vi "DAQ setting.vi"(8 "error in (no error)":errorcluster, 11 "vi reference":refnum<vi>) -> (0 "error Out":errorcluster, 3 "Out reference":refnum<vi>)   [LabVIEW 2015]
uses:
  Control Button/Exit.ctl
  Control Button/Save.ctl
  <vilib>/addons/database/Connection.llb/DB Tools Open Connec (String).vi
  <vilib>/addons/database/_DB Variant To Data/Database Variant To Data.xnode
  <vilib>/addons/database/NI_Database_API.lvlib
panel:
  out "error out":errorcluster
  in  "read":bool
  out "subarray":string[](array[string])
  in  "Save":T1
  in  "Exit":T2
  in  "Tab Control":T3(tab)
  in  "DAQmx OutPut Setting":T4
  in  "DAQmx InPut Setting":T5
  in  "DAQmx Analog Input Setting":T6
  in  "DAQmx  Counter In":tag
  in  "DAQmx  Counter In":tag
  in  "DAQmx Counter Out":tag
  # "Digital Output  Configuration"
  # "Digital Input Configuration"
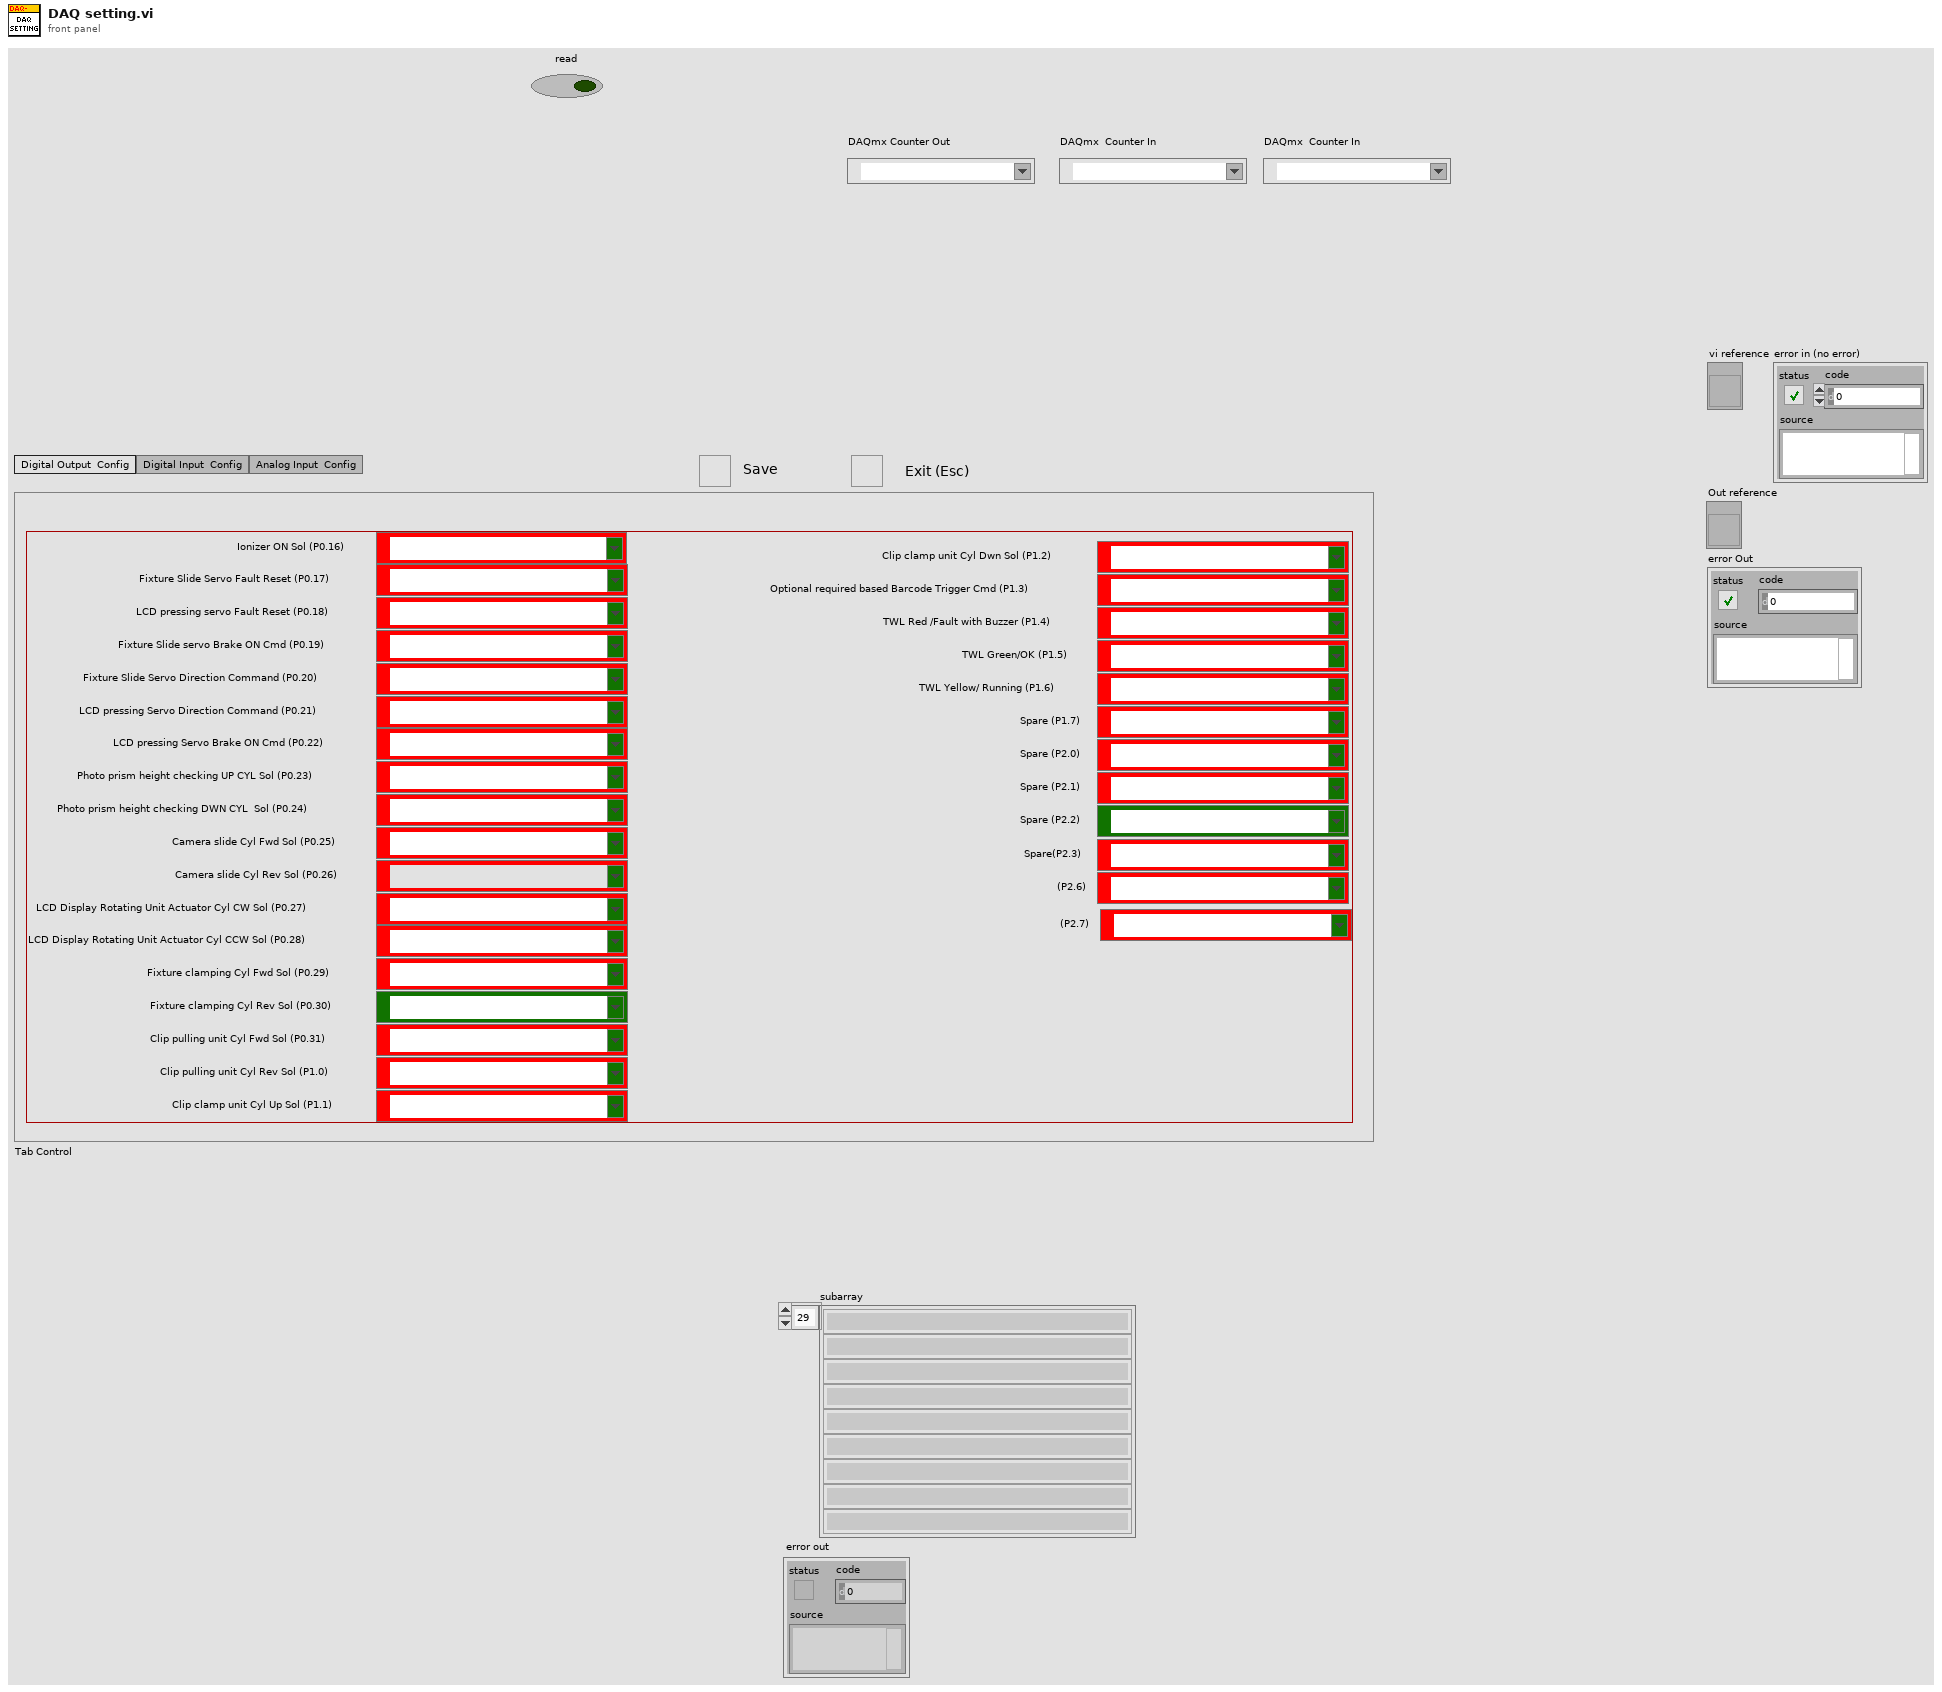
[diagram p1: front panel]
types:
  T1 = typedef "Save.ctl" = bool
  T2 = typedef "Exit.ctl" = bool
  T3 = enum32{"Digital Output  Config", "Digital Input  Config", "Analog Input  Config"}
  T4 = cluster{"DAQmx OutPut_00":tag, "DAQmx OutPut_01":tag, "DAQmx OutPut_02":tag, "DAQmx OutPut_03":tag, "DAQmx OutPut_04":tag, "DAQmx OutPut_05":tag, "DAQmx OutPut_06":tag, "DAQmx OutPut_07":tag, "DAQmx OutPut_08":tag, "DAQmx OutPut_09":tag, "DAQmx OutPut_10":tag, "DAQmx OutPut_11":tag, "DAQmx OutPut_12":tag, "DAQmx OutPut_13":tag, "DAQmx OutPut_14":tag, "DAQmx OutPut_15":tag, "DAQmx OutPut_16":tag, "DAQmx OutPut_17":tag, "DAQmx OutPut_18":tag, "DAQmx OutPut_19":tag, "DAQmx OutPut_20":tag, "DAQmx OutPut_21":tag, "DAQmx OutPut_22":tag, "DAQmx OutPut_23":tag, "DAQmx OutPut_12 2":tag, "DAQmx OutPut_13 2":tag, "DAQmx OutPut_14 2":tag, "DAQmx OutPut_15 2":tag, "DAQmx OutPut_16 2":tag, "String":string, "DAQmx OutPut_16 3":tag}
  T5 = cluster{"DAQmx InPut_00":tag, "DAQmx InPut_01":tag, "DAQmx InPut_02":tag, "DAQmx InPut_03":tag, "DAQmx InPut_04":tag, "DAQmx InPut_05":tag, "DAQmx InPut_06":tag, "DAQmx InPut_07":tag, "DAQmx InPut_08":tag, "DAQmx InPut_09":tag, "DAQmx InPut_10":tag, "DAQmx InPut_11":tag, "DAQmx InPut_12":tag, "DAQmx InPut_13":tag, "DAQmx InPut_14":tag, "DAQmx InPut_15":tag, "Key":string}
  T6 = cluster{"DAQmx Analog Input_00":tag, "DAQmx Analog Input_01":tag, "DAQmx Analog Input_02":tag, "DAQmx Analog Input_03":tag, "DAQmx Analog Input_04":tag, "DAQmx Analog Input_05":tag, "DAQmx Analog Input_06":tag, "DAQmx Analog Input_07":tag, "DAQmx Analog Input_08":tag, "DAQmx Analog Input_09":tag, "DAQmx Analog Input_10":tag, "DAQmx Analog Input_11":tag, "DAQmx Analog Input_12":tag, "DAQmx Analog Input_13":tag, "DAQmx Analog Input_14":tag, "DAQmx Analog Input_15":tag, "DAQmx Analog Input_16":tag, "DAQmx Analog Input_17":tag, "DAQmx Analog Input_18":tag, "DAQmx Analog Input_19":tag, "DAQmx Analog Input_20":tag, "DAQmx Analog Input_21":tag, "DAQmx Analog Input_22":tag, "DAQmx Analog Input_23":tag, "DAQmx Analog Input_24":tag, "DAQmx Analog Input_25":tag, "DAQmx Analog Input_26":tag, "DAQmx Analog Input_27":tag, "DAQmx Analog Input_28":tag, "DAQmx Analog Input_29":tag, "DAQmx Analog Input_30":tag, "DAQmx Analog Input_31":tag, "String 2":string}
  T7 = enum8{"Enabled", "Disabled", "Disabled and Grayed Out"}
  T8 = typedef "NI_Database_API.lvlib/Conn ObjectReference.ctl" = refnum<k1>
  T9 = cluster{"data[0]":string, "data[1]":string, "data[2]":string, "data[3]":string, "data[4]":string, "data[5]":string, "data[6]":string, "data[7]":string, "data[8]":string, "data[9]":string, "data[10]":string, "data[11]":string, "data[12]":string, "data[13]":string, "data[14]":string, "data[15]":string, "data[16]":string}
  T10 = cluster{"data[0]":string, "data[1]":string, "data[2]":string, "data[3]":string, "data[4]":string, "data[5]":string, "data[6]":string, "data[7]":string, "data[8]":string, "data[9]":string, "data[10]":string, "data[11]":string, "data[12]":string, "data[13]":string, "data[14]":string, "data[15]":string, "data[16]":string, "data[17]":string, "data[18]":string, "data[19]":string, "data[20]":string, "data[21]":string, "data[22]":string, "data[23]":string, "data[24]":string, "data[25]":string, "data[26]":string, "data[27]":string, "data[28]":string, "data[29]":string, "data[30]":string}
  T11 = cluster{"data[0]":string, "data[1]":string, "data[2]":string, "data[3]":string, "data[4]":string, "data[5]":string, "data[6]":string, "data[7]":string, "data[8]":string, "data[9]":string, "data[10]":string, "data[11]":string, "data[12]":string, "data[13]":string, "data[14]":string, "data[15]":string, "data[16]":string, "data[17]":string, "data[18]":string, "data[19]":string, "data[20]":string, "data[21]":string, "data[22]":string, "data[23]":string, "data[24]":string, "data[25]":string, "data[26]":string, "data[27]":string, "data[28]":string, "data[29]":string, "data[30]":string, "data[31]":string, "data[32]":string}
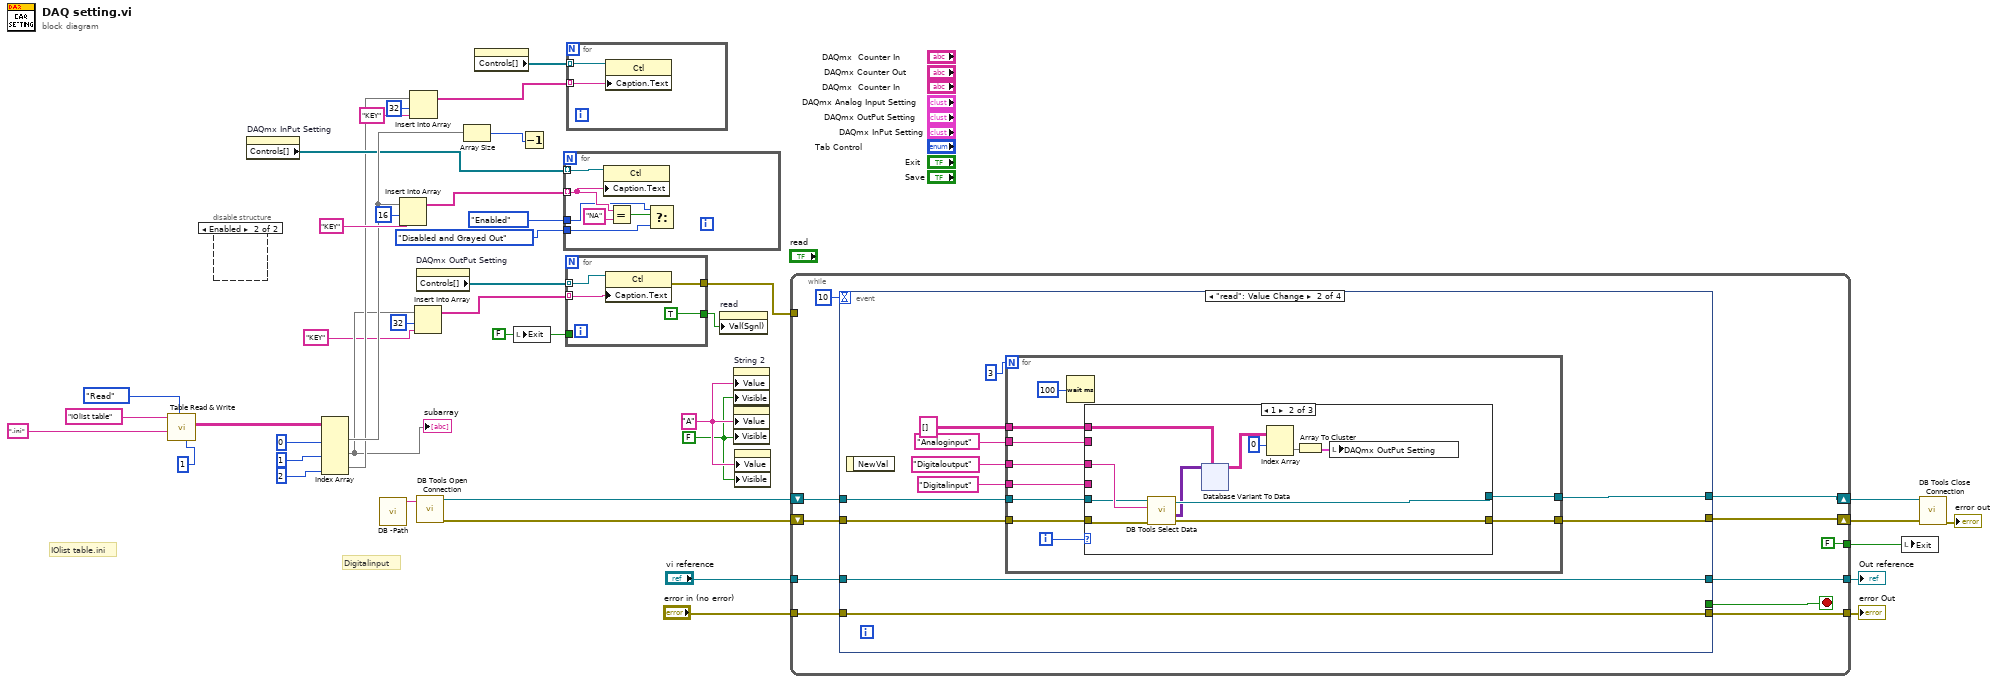
[diagram p0: block diagram]
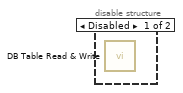
[diagram p2: hidden frame]
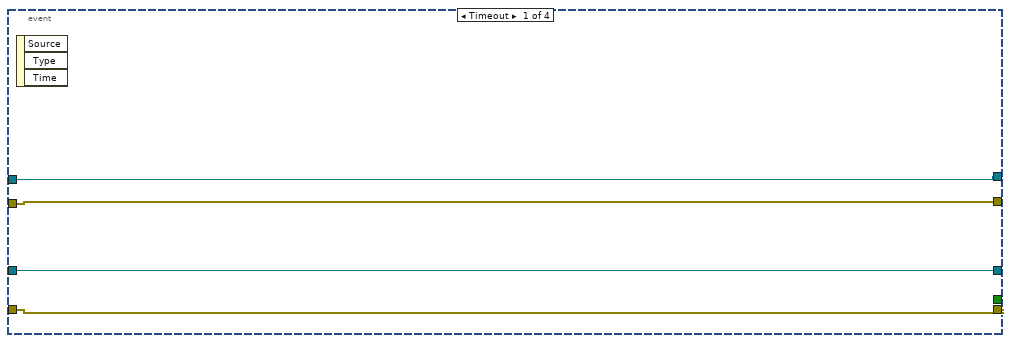
[diagram p3: hidden frame]
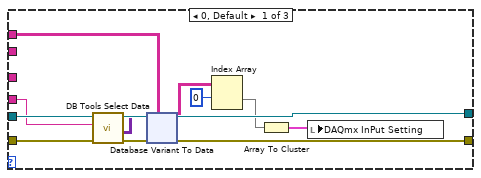
[diagram p4: hidden frame]
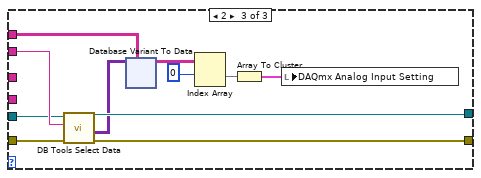
[diagram p5: hidden frame]
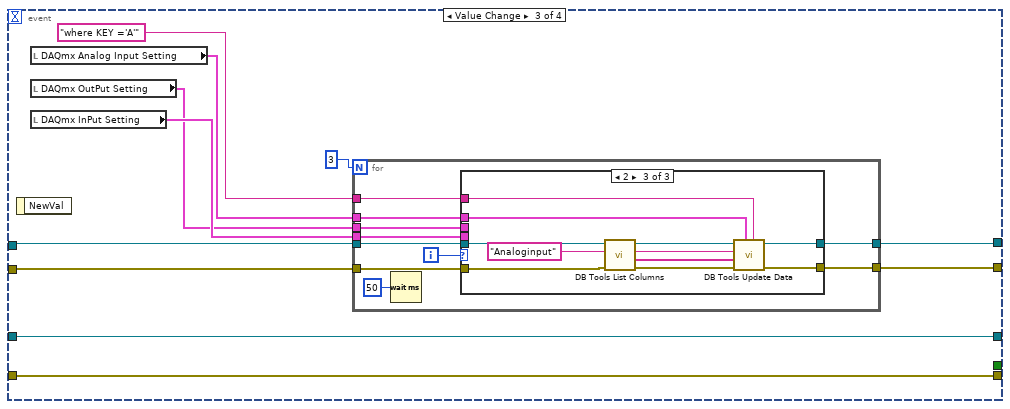
[diagram p6: hidden frame]
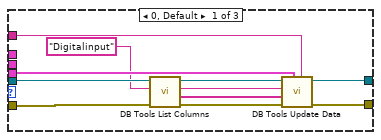
[diagram p7: hidden frame]
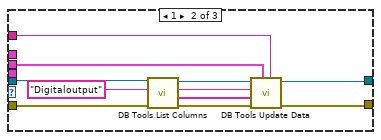
[diagram p8: hidden frame]
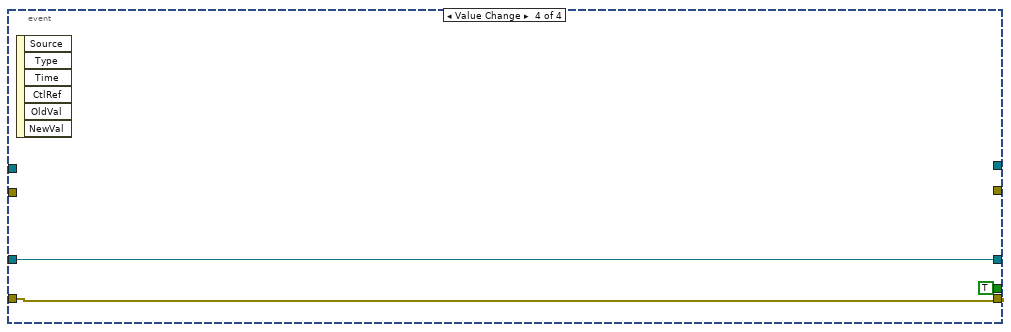
[diagram p9: hidden frame]
diagram:
  w1 = FALSE ("Visible")
  w2 = "A" ("Value")
  w33 = T2 FALSE ("Exit")
  # "IOlist table.ini"
  # "Digitalinput"
  n1 = call "Table Read & Write.vi"("File Name"="IOlist table", "File type"=".ini", "Enum"=enum16{"Read", "Write"}."Read", "index"=1) -> ("Read Table"=w29:string[][])  [unwired: 5 in, 1 out]
  n2 = disable-structure shown="Enabled" {
    frame Disabled {
      n3 = call "DB Table Read & Write.vi"() -> ()  [unwired: 10 in, 2 out]
    }
    frame Enabled {
    }
  }
  n4 = property on="DAQmx InPut Setting" class="Clust (strict)"() -> ("Controls[]"=w12:refnum<vi>[])  [unwired: 2 in, 2 out]
  n5 = Index Array(array=w29, index (col) #1=0 ("disabled index (col)"), index (col) #2=1 ("index (col)"), index (col) #3=2 ("index (col)")) -> (element #1=w14:string[], element #2=w8:string[], element #3=w10:string[])  [unwired: 3 in]
  "subarray" <- w8
  n6 = call "DB -Path.vi"() -> ("String"=w26:string)  [unwired: 11 in]
  n7 = Insert Into Array(array=w14, index=16, new element="KEY" ("new element/subarray")) -> (w13:string[])
  n8 = Insert Into Array(array=w10, index=32, new element="KEY" ("new element/subarray")) -> (w3:string[])
  n9 = Insert Into Array(array=w8, index=32, new element="KEY" ("new element/subarray")) -> (w5:string[])
  n10 = property on="DAQmx OutPut Setting" class="Clust (strict)"() -> ("Controls[]"=w39:refnum<vi>[])  [unwired: 2 in, 2 out]
  n11 = call-poly <vilib>:"DB Tools Open Connection.vi"("connection information"=w26) -> ("error out"=w24:errorcluster, "connection reference"=w25:T8)  [unwired: 7 in]
  n12 = Array Size(array=w14) -> (size(s)=w17:i32)
  n13 = property on="DAQmx Analog Input Setting" class="Clust (strict)"() -> ("Controls[]"=w4:refnum<vi>[])  [unwired: 2 in, 2 out]
  n14 = local write "Exit"(w33) -> ()
  n15 = Decrement(x=w17) -> ()  [unwired: 1 out]
  n16 = for {
    tunnel: w12 -> [w48] mode=indexing
    tunnel: w13 -> [w46] mode=indexing
    tunnel: T7."Enabled" ("Disabled") -> [w45]
    tunnel: T7."Disabled and Grayed Out" ("Disabled") -> [w44]
    n17 = property class="Ctl"(reference=w48, "Caption.Text"=w46) -> ()  [unwired: 1 in, 2 out]
    n18 = Equal?(x=w46, y="NA") -> (x = y?=w43:bool)
    n19 = Select(t=w45, s=w43, f=w44) -> ()  [unwired: 1 out]
  }
  n20 = for {
    tunnel: w39 -> [w52] mode=indexing
    tunnel: w5 -> [w51] mode=indexing
    tunnel: w33 -> [_]
    tunnel: [w50] -> w28
    tunnel: [TRUE] -> w27
    n21 = property class="Ctl"(reference=w52, "Caption.Text"=w51) -> (error out=w50:errorcluster)  [unwired: 1 in, 1 out]
  }
  n22 = for {
    tunnel: w4 -> [w54] mode=indexing
    tunnel: w3 -> [w53] mode=indexing
    n23 = property class="Ctl"(reference=w54, "Caption.Text"=w53) -> ()  [unwired: 1 in, 2 out]
  }
  n24 = property on="read" class="Bool (strict)"("Val(Sgnl)"=w27) -> ()  [unwired: 2 in, 2 out]
  n25 = property on="String 2" class="Str"("Value"=w2, "Visible"=w1) -> ()  [unwired: 2 in, 2 out]
  n26 = property on="Key" class="Str"("Value"=w2, "Visible"=w1) -> ()  [unwired: 2 in, 2 out]
  n27 = property on="String" class="Str"("Value"=w2, "Visible"=w1) -> ()  [unwired: 2 in, 2 out]
  n28 = while {
    tunnel: [FALSE] -> w38
    tunnel: "vi reference" -> [w62]
    tunnel: "error in (no error)" -> [w61]
    tunnel: [w60] -> w35
    tunnel: [w59] -> w34
    tunnel: w28 -> [_]
    shift-right: [w56] -> w23
    shift-left: w25 -> [w58]
    shift-right: [w55] -> w22
    shift-left: w24 -> [w57]
    stop <- w64 stop-if-true
    n29 = event shown="[1] \"read\": Value Change" {
      selector: _ -> [_ _ _ _]
      dyn-events: _ -> [_ _ _ _]
      timeout: 10 -> [_ _ _ _]
      tunnel: [_ _ _ TRUE] -> w64
      tunnel: w62 -> [w69 w80 w267 w309]
      tunnel: w61 -> [w68 w79 w266 w308]
      tunnel: [w69 w80 w267 w309] -> w60
      tunnel: [w68 w79 w266 w308] -> w59
      tunnel: w58 -> [w67 w73 w265 _]
      tunnel: w57 -> [w66 w72 w264 _]
      tunnel: [w67 w75 w262 _] -> w56
      tunnel: [w66 w74 w261 _] -> w55
      event Timeout {
        n30 = event-data() -> ()  [unwired: 1 in, 3 out]
      }
      event "read": Value Change {
        n31 = event-data() -> ()  [unwired: 1 in, 1 out]
        n32 = for {
          N: 3 -> [_]
          tunnel: "Digitalinput" ("table") -> [w88]
          tunnel: w73 -> [w87]
          tunnel: w72 -> [w86]
          tunnel: [w85] -> w75
          tunnel: [w84] -> w74
          tunnel: "Digitaloutput" ("table") -> [w83]
          tunnel: "Analoginput" ("table") -> [w82]
          tunnel: string[][] [] -> [w81]
          i -> [w90]
          n33 = Wait (ms)(milliseconds to wait=u32 100) -> ()  [unwired: 1 out]
          n34 = case shown="1" w90 {
            tunnel: w88 -> [w96 _ _]
            tunnel: w87 -> [w101 w156 w209]
            tunnel: w86 -> [w100 w155 w208]
            tunnel: [w99 w153 w207] -> w85
            tunnel: [w98 w152 w206] -> w84
            tunnel: w83 -> [_ w157 _]
            tunnel: w82 -> [_ _ w211]
            tunnel: w81 -> [w97 w154 w210]
            frame 0, Default {
              n35 = call <vilib>:"DB Tools Select Data.vi"("error in (no error)"=w100, "table"=w96, "connection reference"=w101) -> ("error out"=w91:errorcluster, "data"=w95:variant[][], "connection reference out"=w99:T8)  [unwired: 3 in]
              n36 = xnode "Database Variant To Data"("database variant"=w95, "error in (no error)"=w91, "type"=w97) -> ("data"=w94:string[][], "error out"=w98:errorcluster)
              n37 = Index Array(array=w94, index (row)=0) -> (element=w93:string[])  [unwired: 1 in]
              n38 = Array To Cluster(array=w93) -> (cluster=w92:T9)
              n39 = local write "DAQmx InPut Setting"(w92) -> ()
            }
            frame 1 {
              n40 = call <vilib>:"DB Tools Select Data.vi"("error in (no error)"=w155, "table"=w157, "connection reference"=w156) -> ("error out"=w152:errorcluster, "data"=w151:variant[][], "connection reference out"=w153:T8)  [unwired: 3 in]
              n41 = xnode "Database Variant To Data"("database variant"=w151, "type"=w154) -> ("data"=w150:string[][])  [unwired: 1 in, 1 out]
              n42 = Index Array(array=w150, index (row)=0 ("disabled index (col)")) -> (element=w148:string[])  [unwired: 1 in]
              n43 = Array To Cluster(array=w148) -> (cluster=w147:T10)
              n44 = local write "DAQmx OutPut Setting"(w147) -> ()
            }
            frame 2 {
              n45 = call <vilib>:"DB Tools Select Data.vi"("error in (no error)"=w208, "table"=w211, "connection reference"=w209) -> ("error out"=w206:errorcluster, "data"=w204:variant[][], "connection reference out"=w207:T8)  [unwired: 3 in]
              n46 = xnode "Database Variant To Data"("database variant"=w204, "type"=w210) -> ("data"=w205:string[][])  [unwired: 1 in, 1 out]
              n47 = Index Array(array=w205, index (row)=0 ("disabled index (col)")) -> (element=w203:string[])  [unwired: 1 in]
              n48 = Array To Cluster(array=w203) -> (cluster=w202:T11)
              n49 = local write "DAQmx Analog Input Setting"(w202) -> ()
            }
          }
        }
      }
      event Value Change {
        n50 = event-data() -> ()  [unwired: 1 in, 1 out]
        n51 = local read "DAQmx Analog Input Setting"() -> (w258:T6)
        n52 = local read "DAQmx OutPut Setting"() -> (w257:T4)
        n53 = local read "DAQmx InPut Setting"() -> (w263:T5)
        n54 = for {
          N: 3 -> [_]
          tunnel: w265 -> [w276]
          tunnel: w264 -> [w275]
          tunnel: w258 -> [w274]
          tunnel: w257 -> [w273]
          tunnel: w263 -> [w272]
          tunnel: [w271] -> w262
          tunnel: [w270] -> w261
          tunnel: "where KEY ='A'" -> [w268]
          i -> [w277]
          n55 = Wait (ms)(milliseconds to wait=u32 50) -> ()  [unwired: 1 out]
          n56 = case shown="2" w277 {
            tunnel: w276 -> [w284 w293 w307]
            tunnel: w275 -> [w283 w294 w302]
            tunnel: w274 -> [_ _ w304]
            tunnel: w273 -> [_ w295 _]
            tunnel: w272 -> [w285 _ _]
            tunnel: [w287 w297 w306] -> w271
            tunnel: [w286 w296 w305] -> w270
            tunnel: w268 -> [w278 w288 w298]
            frame 0, Default {
              w279 = "Digitalinput" ("table")
              n57 = call <vilib>:"DB Tools List Columns.vi"("error in (no error)"=w283, "table"=w279, "connection reference"=w284) -> ("error out"=w280:errorcluster, "columns"=w282:string[], "connection reference out"=w281:T8)  [unwired: 1 in, 1 out]
              n58 = call <vilib>:"DB Tools Update Data.vi"("condition"=w278, "data"=w285, "error in (no error)"=w280, "columns"=w282, "table"=w279, "connection reference"=w281) -> ("error out"=w286:errorcluster, "connection reference out"=w287:T8)  [unwired: 4 in]
            }
            frame 1 {
              w289 = "Digitaloutput" ("table")
              n59 = call <vilib>:"DB Tools List Columns.vi"("error in (no error)"=w294, "table"=w289, "connection reference"=w293) -> ("error out"=w292:errorcluster, "columns"=w290:string[], "connection reference out"=w291:T8)  [unwired: 1 in, 1 out]
              n60 = call <vilib>:"DB Tools Update Data.vi"("condition"=w288, "data"=w295, "error in (no error)"=w292, "columns"=w290, "table"=w289, "connection reference"=w291) -> ("error out"=w296:errorcluster, "connection reference out"=w297:T8)  [unwired: 4 in]
            }
            frame 2 {
              w300 = "Analoginput" ("table")
              n61 = call <vilib>:"DB Tools List Columns.vi"("error in (no error)"=w302, "table"=w300, "connection reference"=w307) -> ("error out"=w301:errorcluster, "columns"=w299:string[], "connection reference out"=w303:T8)  [unwired: 1 in, 1 out]
              n62 = call <vilib>:"DB Tools Update Data.vi"("condition"=w298, "data"=w304, "error in (no error)"=w301, "columns"=w299, "table"=w300, "connection reference"=w303) -> ("error out"=w305:errorcluster, "connection reference out"=w306:T8)  [unwired: 4 in]
            }
          }
        }
      }
      event Value Change {
        n63 = event-data() -> ()  [unwired: 1 in, 6 out]
      }
    }
  }
  "Out reference" <- w35
  "error Out" <- w34
  n64 = local write "Exit"(w38) -> ()
  n65 = call <vilib>:"DB Tools Close Connection.vi"("error in (no error)"=w22, "connection reference"=w23) -> ("error out"=→"error out":errorcluster)  [unwired: 5 in]
